vi "Vi_CreationDesSequences.vi"(4 "Go2":bool, 5 "Angle X":dbl, 6 "Go1":bool, 7 "Vitesse X":dbl, 8 "stop moteurs":bool, 9 "Vitesse Y":dbl, 10 "Enregistrer sequence X":bool, 11 "Angle Y":dbl) -> (1 "Deverouillé":bool, 2 "Connecté":bool, 3 "Sequence":T1)   [LabVIEW 2015]
uses:
  Variable globale.vi
  <userlib>/ICNC/ICNC2.lvlib
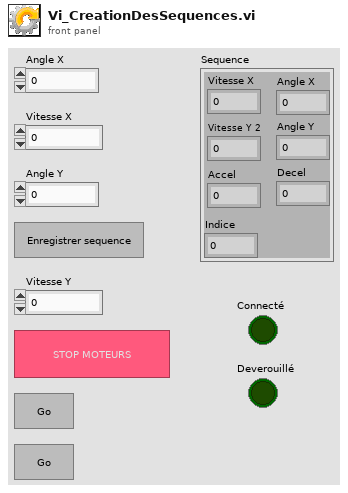
[diagram p1: front panel]
types:
  T1 = cluster{"Angle X":dbl, "Vitesse X":dbl, "Angle Y":dbl, "Accel":dbl, "Decel":dbl, "Indice":dbl, "Vitesse Y 2":dbl}
  T2 = cluster{"Angle X":dbl, "Vitesse X":dbl, "Angle Y":dbl, "Vitesse Y":dbl, "Accel":dbl, "Decel":dbl, dbl}
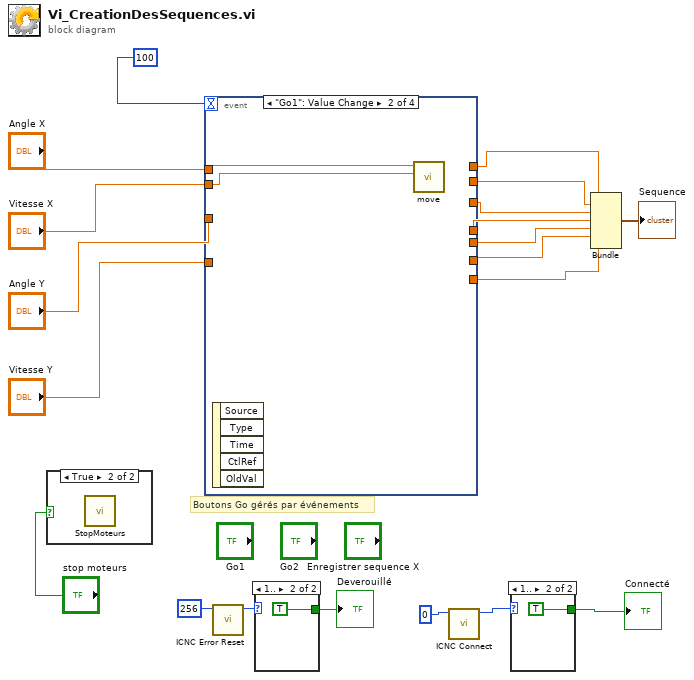
[diagram p0: block diagram]
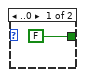
[diagram p2: hidden frame]
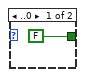
[diagram p3: hidden frame]
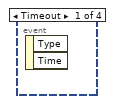
[diagram p5: hidden frame]
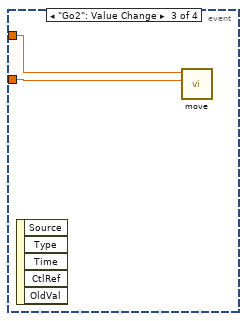
[diagram p6: hidden frame]
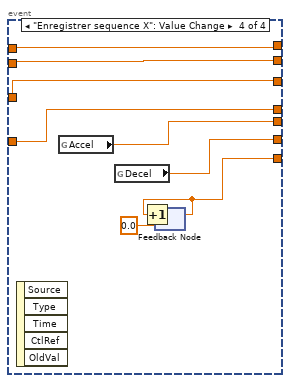
[diagram p7: hidden frame]
diagram:
  # "Boutons Go gérés par événements"
  n1 = case shown="True" "stop moteurs" {
    frame False {
    }
    frame True {
      n2 = call "StopMoteurs.vi"() -> ()  [unwired: 12 in]
    }
  }
  n3 = event shown="[1] \"Go1\": Value Change" {
    selector: _ -> [_ _ _ _]
    dyn-events: _ -> [_ _ _ _]
    timeout: 100 -> [_ _ _ _]
    tunnel: "Angle X" -> [_ w22 _ w33]
    tunnel: "Vitesse X" -> [_ w21 _ w32]
    tunnel: "Angle Y" -> [_ _ w23 w26]
    tunnel: "Vitesse Y" -> [_ _ w24 w25]
    tunnel: [_ _ _ w33] -> w13
    tunnel: [_ _ _ w32] -> w14
    tunnel: [_ _ _ w30] -> w19
    tunnel: [_ _ _ w28] -> w17
    tunnel: [_ _ _ w27] -> w18
    tunnel: [_ _ _ w26] -> w15
    tunnel: [_ _ _ w25] -> w16
    event Timeout {
      n4 = event-data() -> ()  [unwired: 1 in, 2 out]
    }
    event "Go1": Value Change {
      n5 = event-data() -> ()  [unwired: 1 in, 5 out]
      n6 = call "move.vi"("Vitesse"=w21, "Angle"=w22) -> ()  [unwired: 10 in]
    }
    event "Go2": Value Change {
      n7 = event-data() -> ()  [unwired: 1 in, 5 out]
      n8 = call "move.vi"("Vitesse"=w24, "Angle"=w23) -> ()  [unwired: 10 in]
    }
    event "Enregistrer sequence X": Value Change {
      n9 = event-data() -> ()  [unwired: 1 in, 5 out]
      n10 = global read "Variable globale.vi" "Accel"() -> (w28:dbl)
      n11 = global read "Variable globale.vi" "Decel"() -> (w27:dbl)
      n12 = feedback #1(0.0) -> (w30:dbl)
      n13 = Increment(x=w30) -> (x+1=w31:dbl)
      n14 = feedback-in #1(w31) -> ()
    }
  }
  n15 = call <userlib>:"ICNC Error Reset.vi"("ErrorBits"=256) -> ("function return"=w5:u32)  [unwired: 9 in, 1 out]
  n16 = case shown="1.." w5 {
    tunnel: [FALSE TRUE] -> w2
    frame ..0 {
    }
    frame 1.. {
    }
  }
  "Deverouillé" <- w2
  n17 = call <userlib>:"ICNC Connect.vi"("ICNC_Number"=0) -> ("function return"=w4:u32)  [unwired: 9 in, 1 out]
  n18 = case shown="1.." w4 {
    tunnel: [FALSE TRUE] -> w1
    frame ..0 {
    }
    frame 1.. {
    }
  }
  "Connecté" <- w1
  n19 = Bundle("Angle X"=w13, "Vitesse X"=w14, "Angle Y"=w15, "Vitesse Y"=w16, "Accel"=w17, "Decel"=w18, w19) -> (→"Sequence":T2)  [unwired: 1 in]
